vi "WPI_Power Set roboRIO Rail Disable.vi"(5 "Disable User 3.3 V Rail":bool, 7 "Disable User 5V Rail":bool, 9 "Disable User 6V Rail":bool, 11 "error in":errorcluster) -> (15 "error out":errorcluster)   [LabVIEW 2017]
doc: "Provides the ability to disable user rail voltages on the roboRIO."
uses:
  <vilib>/Utility/error.llb/Error Cluster From Error Code.vi
  <vilib>/rvi/errors/niLvFpgaAdjustHostInterfaceError.vi
  <vilib>/rvi/interface/nirviReadWriteControl/nirviReadWriteControl.xnode
  <vilib>/Rock Robotics/SystemInterfaces/System/FPGA_SystemFRC FPGA Ref.ctl
  NiFpgaLv.dll
  <vilib>/rvi/interface/Simulation/niFpgaSimulationCallBeginRW.vi
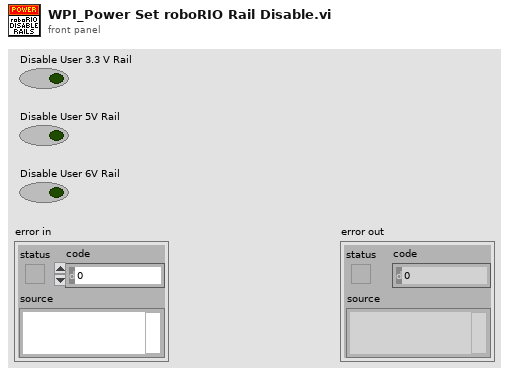
[diagram p1: front panel]
types:
  T1 = cluster{"User3V3":bool, "User5V":bool, "User6V":bool}
  T2 = typedef "FPGA_SystemFRC FPGA Ref.ctl" = refnum<k20>
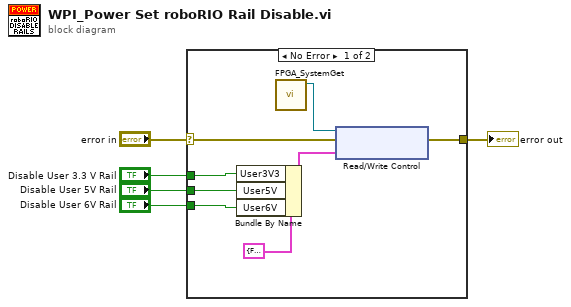
[diagram p0: block diagram]
diagram:
  n1 = case shown="No Error" "error in" {
    selector: "error in" -> [w12 w14]
    tunnel: [w11 w14] -> w4
    tunnel: "Disable User 3.3 V Rail" -> [w8 _]
    tunnel: "Disable User 5V Rail" -> [w7 _]
    tunnel: "Disable User 6V Rail" -> [w6 _]
    frame No Error {
      n2 = Bundle By Name(cluster=T1 {"User3V3"=FALSE, "User5V"=FALSE, "User6V"=FALSE} ("Power.Disable"), "User3V3"=w8, "User5V"=w7, "User6V"=w6) -> (w9:T1)
      n3 = call <vilib>:"FPGA_SystemGet.vi"() -> ("FRC FPGA Ref"=w13:T2)  [unwired: 2 in, 9 out]
      n4 = xnode "Read/Write Control"("FPGA VI Reference In"=w13, "error in"=w12, "Power.Disable"=w9) -> ("error out"=w11:errorcluster)  [unwired: 1 out]
    }
    frame Error {
    }
  }
  "error out" <- w4
